vi "Read Position.vi"(2 "error in (no error)":errorcluster, 3 "Sensor.lvclass":refnum<class "Sensor.lvclass">) -> (0 "error out":errorcluster, 1 "Position":dbl[](array[numeric]))   [LabVIEW 2015, in "Sensor.lvclass"]
uses:
  Sensor.lvclass
  Sensor.lvclass/Sensor.ctl
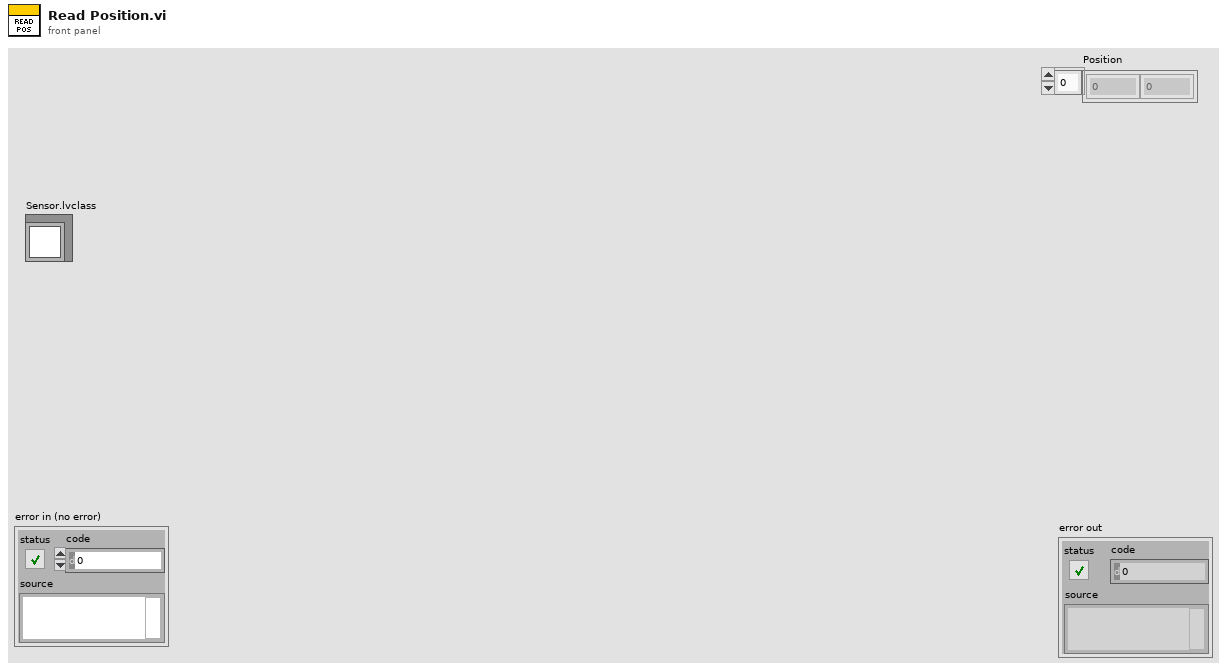
[diagram p1: front panel]
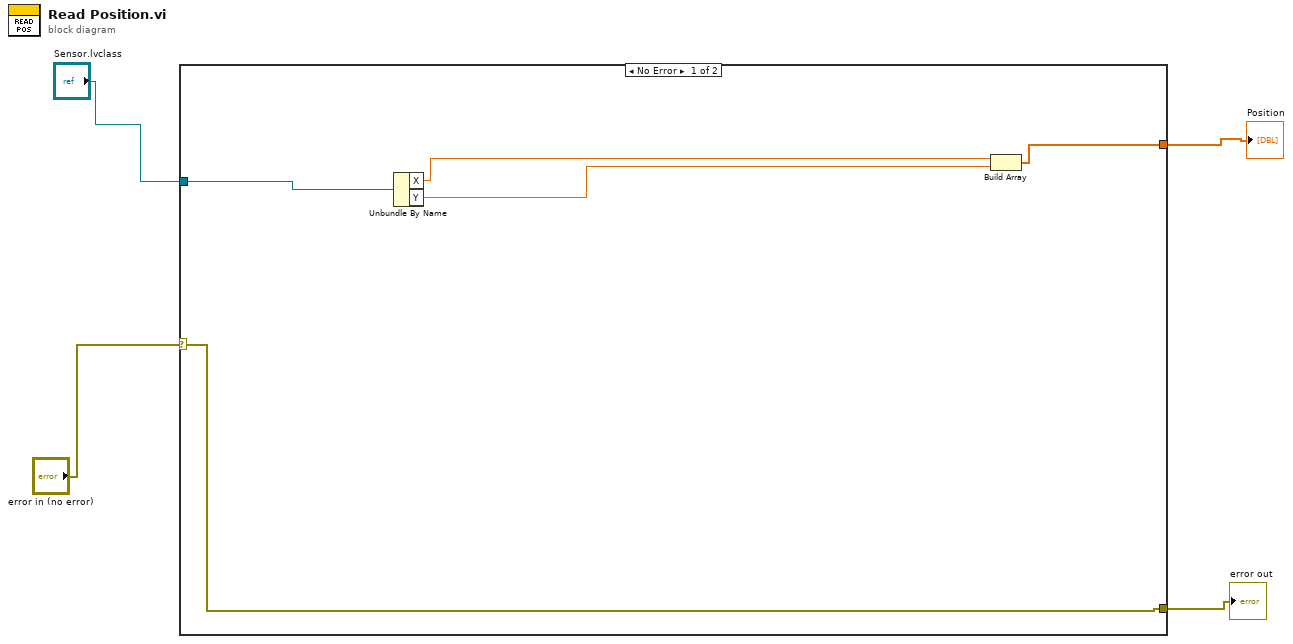
[diagram p0: block diagram]
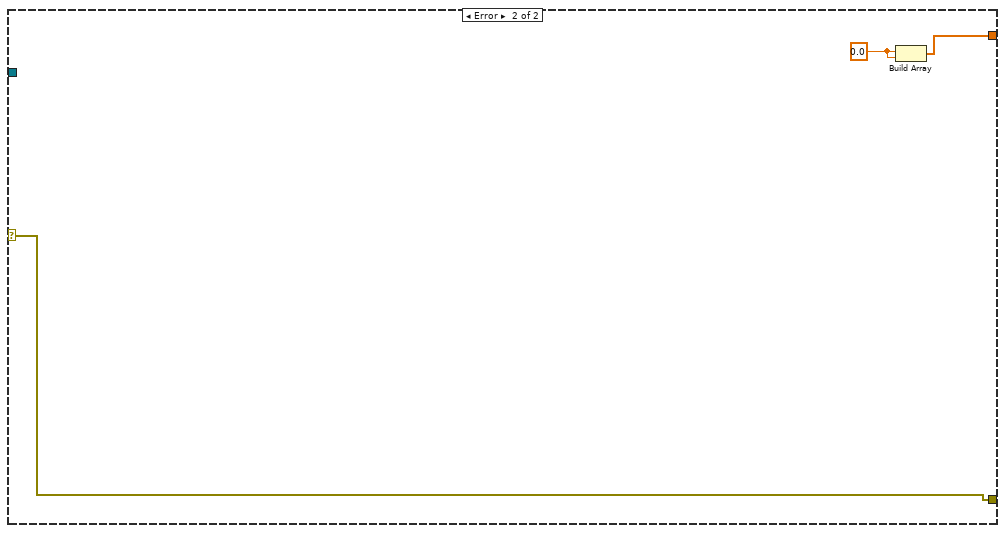
[diagram p2: hidden frame]
diagram:
  n1 = case shown="No Error" "error in (no error)" {
    selector: "error in (no error)" -> [w9 w11]
    tunnel: [w9 w11] -> w3
    tunnel: [w5 w10] -> w2
    tunnel: "Sensor.lvclass" -> [w8 _]
    frame No Error {
      n2 = Unbundle By Name(w8) -> ("X"=w7:dbl, "Y"=w6:dbl)
      n3 = Build Array(w7, w6) -> (w5:dbl[])
    }
    frame Error {
      w12 = 0.0
      n4 = Build Array(w12, w12) -> (w10:dbl[])
    }
  }
  "error out" <- w3
  "Position" <- w2
